vi "PH_Connection.VISA get Information.vi"(5 "error in":errorcluster) -> (16 "VISA Information":T1(array[cluster]) {"Interface Information: Interface Type" items=["GPIB"=1, "VXI"=2, "GPIB-VXI"=3, "Serial"=4, "PXI"=5, "TCPIP"=6, "USB"=7, "FireWire"=9]}, 19 "error out":errorcluster)   [LabVIEW 2014, in "PH_Common.lvlib"]
uses:
  PH_Common.lvlib
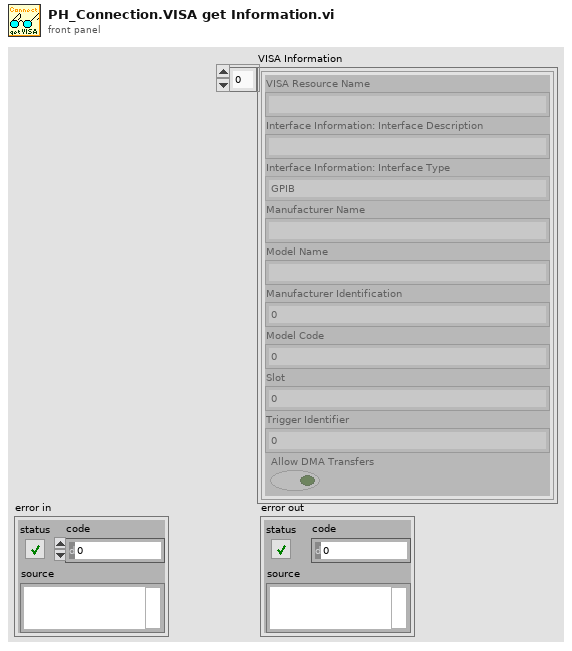
[diagram p1: front panel]
types:
  T1 = cluster{"VISA Resource Name":string, "Interface Information: Interface Description":string, "Interface Information: Interface Type":u16, "Manufacturer Name":string, "Model Name":string, "Manufacturer Identification":u16, "Model Code":u16, "Slot":i16, "Trigger Identifier":i16, "Allow DMA Transfers":bool}[]
  T2 = cluster{"VISA Resource Name":string, "Interface Information: Interface Description":string, "Interface Information: Interface Type":u16, "Manufacturer Name":string, "Model Name":string, "Manufacturer Identification":u16, "Model Code":u16, "Slot":i16, "Trigger Identifier":i16, "Allow DMA Transfers":bool}
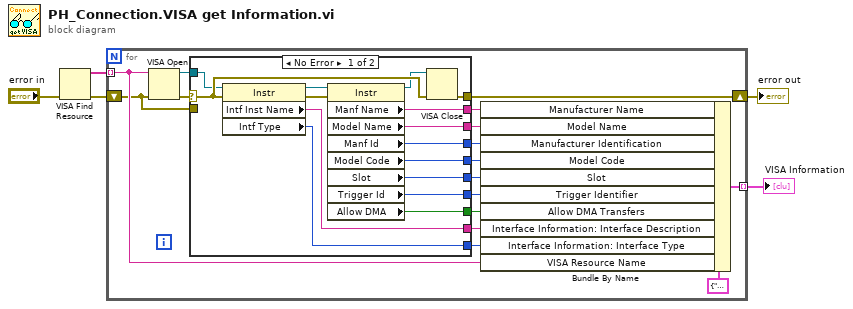
[diagram p0: block diagram]
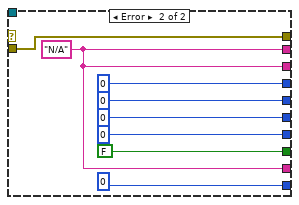
[diagram p2: hidden frame]
diagram:
  n1 = VISA Find Resource(8:"error in") -> (0:w2:errorcluster, 3:w3:string[])  [unwired: 2 in, 1 out]
  n2 = for {
    shift-right: [w21] -> w4
    shift-left: w2 -> [w10]
    tunnel: w3 -> [w11] mode=indexing
    tunnel: [w13] -> w1 mode=indexing
    n3 = VISA Open(error in (no error)=w10, VISA resource name=w11) -> (VISA resource name=w9:refnum<visa-resource-name>, error out=w12:errorcluster)  [unwired: 3 in]
    n4 = case shown="No Error" w12 {
      selector: w12 -> [w27 _]
      tunnel: [w35 w43] -> w21
      tunnel: w9 -> [w26 _]
      tunnel: [w28 w37] -> w20
      tunnel: [w34 w37] -> w19
      tunnel: [w33 u16 0 ("Manf Id")] -> w18
      tunnel: [w32 u16 0 ("Model Code")] -> w17
      tunnel: [w31 i16 0 ("Slot")] -> w16
      tunnel: [w30 i16 0 ("Trigger Id")] -> w15
      tunnel: [w29 FALSE ("Allow DMA")] -> w14
      tunnel: w10 -> [_ w43]
      tunnel: [w23 w37] -> w7
      tunnel: [w22 u16 0 ("Intf Type")] -> w6
      frame No Error {
        n5 = property class="Instr"(reference=w26, error in=w27) -> (reference out=w25:refnum<visa-resource-name>, "Intf Inst Name"=w23:string, "Intf Type"=w22:u16)  [unwired: 1 out]
        n6 = property class="Instr"(reference=w25, error in=w27) -> (reference out=w24:refnum<visa-resource-name>, "Manf Name"=w28:string, "Model Name"=w34:string, "Manf Id"=w33:u16, "Model Code"=w32:u16, "Slot"=w31:i16, "Trigger Id"=w30:i16, "Allow DMA"=w29:bool)  [unwired: 1 out]
        n7 = VISA Close(VISA resource name=w24, error in (no error)=w27) -> (error out=w35:errorcluster)
      }
      frame Error {
        w37 = "N/A" ("Manf Name")
      }
    }
    n8 = Bundle By Name(cluster=T2 {"VISA Resource Name"="TCPIP0::140.181.83.202::inst0::INSTR", "Interface Information: Interface Description"="TCPIP0  (LAN <-> PCSPC029.campus.gsi.de)", "Interface Information: Interface Type"=1, "Manufacturer Name"="N/A", "Model Name"="N/A", "Manufacturer Identification"=0, "Model Code"=0, "Slot"=0, "Trigger Identifier"=0, "Allow DMA Transfers"=FALSE} ("Settings"), "Manufacturer Name"=w20, "Model Name"=w19, "Manufacturer Identification"=w18, "Model Code"=w17, "Slot"=w16, "Trigger Identifier"=w15, "Allow DMA Transfers"=w14, "Interface Information: Interface Description"=w7, "Interface Information: Interface Type"=w6, "VISA Resource Name"=w11) -> (w13:T2)
  }
  "VISA Information" <- w1
  "error out" <- w4
